vi "_Validate Tune Property.vi"(6 "ConfigRow #":i32, 7 "User Value":dbl=1.0, 8 "Method In":T1={"Lenses"=[], "Mass Ranges"=[], "Acquire"=FALSE, "MCA"=FALSE, "Q1DC EN"=FALSE, "Q1 POL"=FALSE, "Q3 POL"=FALSE, "Q1 RF  EN"=FALSE, "Averaging"=FALSE, "Log Scale"=FALSE, "CPS"=FALSE, "Unit"=FALSE, "Data Path"=path "", "Run Mode"=enum."MRM (Q1/Q2)", "Fixed Mass (amu)"=1.0, "Q3DC EN"=FALSE, "Q3 RF  EN"=FALSE, "Negative"=FALSE} {"Mass Ranges"."Res" items=["High/High", "Medium/Medium", "Low/Low", "High/Medium", "High/Low", "Medium/High", "Medium/Low", "Low/High", "Low/Medium"]}) -> (0 "Lens Table":string[][](table), 1 "DAC Value Out":i32=1, 2 "User Value Out":dbl=1.0, 3 "Method Out":T1={"Lenses"=[], "Mass Ranges"=[], "Acquire"=FALSE, "MCA"=FALSE, "Q1DC EN"=FALSE, "Q1 POL"=FALSE, "Q3 POL"=FALSE, "Q1 RF  EN"=FALSE, "Averaging"=FALSE, "Log Scale"=FALSE, "CPS"=FALSE, "Unit"=FALSE, "Data Path"=path "", "Run Mode"=enum."MRM (Q1/Q2)", "Fixed Mass (amu)"=1.0, "Q3DC EN"=FALSE, "Q3 RF  EN"=FALSE, "Negative"=FALSE} {"Mass Ranges"."Res" items=["High/High", "Medium/Medium", "Low/Low", "High/Medium", "High/Low", "Medium/High", "Medium/Low", "Low/High", "Low/Medium"]})   [LabVIEW 2012]
uses:
  Type/_GUI Method.ctl
  Type/_Lens Property.ctl
  Type/_Mass Range Property.ctl
  Type/_Mass Range Parameters.ctl
  Type/_RT Res Type.ctl
  Type/_Run Mode.ctl
  _Global Configuration.vi
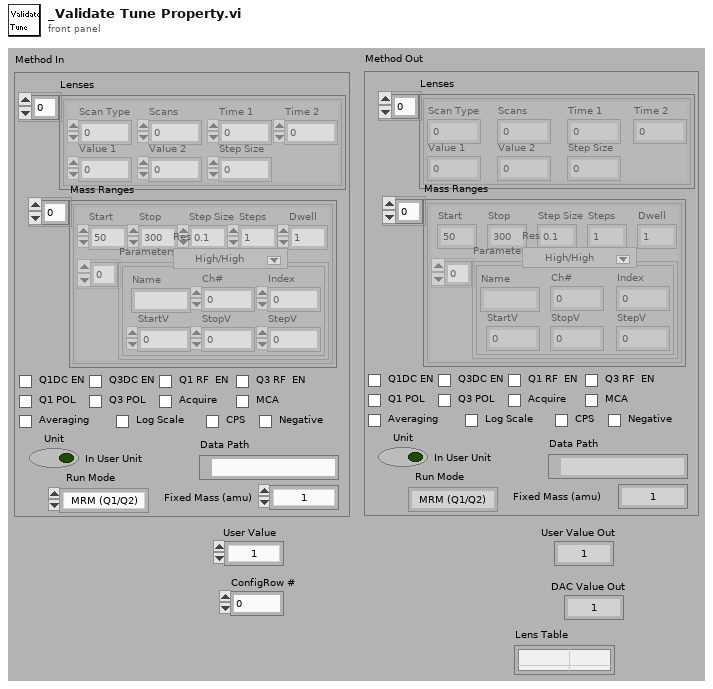
[diagram p1: front panel]
types:
  T1 = typedef "_GUI Method.ctl" = cluster{"Lenses":T2[], "Mass Ranges":T3[], "Acquire":bool, "MCA":bool, "Q1DC EN":bool, "Q1 POL":bool, "Q3 POL":bool, "Q1 RF  EN":bool, "Averaging":bool, "Log Scale":bool, "CPS":bool, "Unit":bool, "Data Path":path, "Run Mode":T6, "Fixed Mass (amu)":dbl, "Q3DC EN":bool, "Q3 RF  EN":bool, "Negative":bool}
  T2 = typedef "_Lens Property.ctl" = cluster{"Scan Type":u8, "Scans":i32, "Time 1":dbl, "Time 2":dbl, "Value 1":dbl, "Value 2":dbl, "Step Size":dbl}
  T3 = typedef "_Mass Range Property.ctl" = cluster{"Start":dbl, "Stop":dbl, "Step Size":dbl, "Steps":i32, "Dwell":dbl, "Parameters":T4[], "Res":T5}
  T4 = typedef "_Mass Range Parameters.ctl" = cluster{"Name":string, "Ch#":u8, "StartV":dbl, "StopV":dbl, "StepV":dbl, "Index":u8}
  T5 = typedef "_RT Res Type.ctl" = u16
  T6 = typedef "_Run Mode.ctl" = enum16{"MRM (Q1/Q2)", "Q1 Scan", "Q1 SRM", "Q2 Scan", "Q2 SRM", "Product Scan", "Precursor Scan", "Neutral Loss", "Neutral Gain"}
  T7 = typedef "_RT Instrument 2.ctl" = cluster{"Table":T8[], "Instrument":string[]}
  T8 = typedef "_RT Configuration 2.ctl" = cluster{"Name":string, "Ch#":u8, "Min":dbl, "Max":dbl, "Def+":dbl, "Def-":dbl, "Offset":dbl, "Slope":dbl, "Type":u8, "Description":string, "SettleT":dbl}
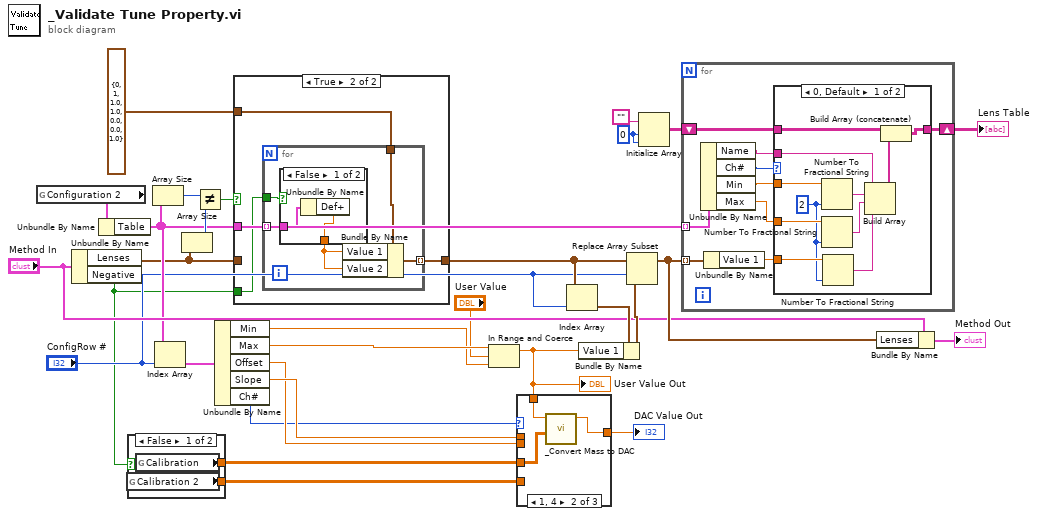
[diagram p0: block diagram]
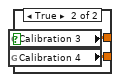
[diagram p2: hidden frame]
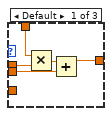
[diagram p3: hidden frame]
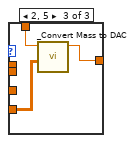
[diagram p4: hidden frame]
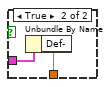
[diagram p6: hidden frame]
diagram:
  w7 = 0 ("dimension size")
  n1 = global read "_Global Configuration.vi" "Configuration 2"() -> (w25:T7)
  n2 = Unbundle By Name("Method In") -> ("Lenses"=w14:T2[], "Negative"=w1:bool)
  n3 = Unbundle By Name(w25) -> ("Table"=w15:T8[])
  n4 = case shown="False" w1 {
    tunnel: [w32 w34] -> w4
    tunnel: [w31 w33] -> w3
    frame False {
      n5 = global read "_Global Configuration.vi" "Calibration 2"() -> (w31:dbl[][])
      n6 = global read "_Global Configuration.vi" "Calibration"() -> (w32:dbl[][])
    }
    frame True {
      n7 = global read "_Global Configuration.vi" "Calibration 3"() -> (w34:dbl[][])
      n8 = global read "_Global Configuration.vi" "Calibration 4"() -> (w33:dbl[][])
    }
  }
  n9 = Array Size(array=w15) -> (size(s)=w18:i32)
  n10 = Index Array(array=w15, index="ConfigRow #") -> (element=w24:T8)
  n11 = Array Size(array=w14) -> (size(s)=w19:i32)
  n12 = Not Equal?(x=w18, y=w19) -> (x != y?=w17:bool)
  n13 = Unbundle By Name(w24) -> ("Min"=w27:dbl, "Max"=w28:dbl, "Offset"=w29:dbl, "Slope"=w30:dbl, "Ch#"=w26:u8)
  n14 = case shown="True" w17 {
    tunnel: w15 -> [_ w39]
    tunnel: w14 -> [w35 _]
    tunnel: [w35 w38] -> w13
    tunnel: T2 {"Scan Type"=0, "Scans"=1, "Time 1"=1.0, "Time 2"=1.0, "Value 1"=0.0, "Value 2"=0.0, "Step Size"=1.0} ("Lenses") -> [_ w37]
    tunnel: w1 -> [_ w36]
    frame False {
    }
    frame True {
      n15 = for {
        tunnel: w39 -> [w43] mode=indexing
        tunnel: w37 -> [w44]
        tunnel: [w41] -> w38 mode=indexing
        tunnel: w36 -> [w40]
        n16 = case shown="False" w40 {
          tunnel: w43 -> [w46 w48]
          tunnel: [w45 w47] -> w42
          frame False {
            n17 = Unbundle By Name(w46) -> ("Def+"=w45:dbl)
          }
          frame True {
            n18 = Unbundle By Name(w48) -> ("Def-"=w47:dbl)
          }
        }
        n19 = Bundle By Name(cluster=w44, "Value 1"=w42, "Value 2"=w42) -> (w41:T2)
      }
    }
  }
  n20 = In Range and Coerce(upper limit=w28, x="User Value", lower limit=w27) -> (coerced(x)=w9:dbl)  [unwired: 1 out]
  "User Value Out" <- w9
  n21 = case shown="1, 4" w26 {
    tunnel: w9 -> [w52 w56 w59]
    tunnel: [w49 w55 w58] -> w10
    tunnel: w30 -> [w51 _ _]
    tunnel: w29 -> [w50 _ _]
    tunnel: w4 -> [_ w54 _]
    tunnel: w3 -> [_ _ w57]
    frame Default {
      n22 = Multiply(x=w52, y=w51) -> (x*y=w53:dbl)
      n23 = Add(x=w53, y=w50) -> (x+y=w49:dbl)
    }
    frame 1, 4 {
      n24 = call "_Convert Mass to DAC.vi"("Calibration Table"=w54, "Mass"=w56) -> ("DAC Value"=w55:dbl)  [unwired: 2 in, 3 out]
    }
    frame 2, 5 {
      n25 = call "_Convert Mass to DAC.vi"("Calibration Table"=w57, "Mass"=w59) -> ("DAC Value"=w58:dbl)  [unwired: 2 in, 3 out]
    }
  }
  "DAC Value Out" <- w10
  n26 = Index Array(array=w13, index="ConfigRow #") -> (element=w23:T2)
  n27 = Bundle By Name(cluster=w23, "Value 1"=w9) -> (w22:T2)
  n28 = Replace Array Subset(array=w13, new element=w22, index="ConfigRow #") -> (w21:T2[])
  n29 = Initialize Array("", w7, w7) -> (w8:string[][])
  n30 = for {
    tunnel: w21 -> [w65] mode=indexing
    tunnel: w15 -> [w66] mode=indexing
    shift-right: [w60] -> w5
    shift-left: w8 -> [w61]
    n31 = Unbundle By Name(w66) -> ("Name"=w63:string, "Ch#"=w62:u8, "Min"=w67:dbl, "Max"=w68:dbl)
    n32 = Unbundle By Name(w65) -> ("Value 1"=w64:dbl)
    n33 = case shown="0, Default" w62 {
      tunnel: w68 -> [w79 _]
      tunnel: w67 -> [w78 _]
      tunnel: [w69 w80] -> w60
      tunnel: w64 -> [w75 _]
      tunnel: w63 -> [w72 _]
      tunnel: w61 -> [w71 w80]
      frame 0, Default {
        w74 = 2
        n34 = Number To Fractional String(number=w78, precision (6)=w74) -> (F-format string=w73:string)  [unwired: 2 out]
        n35 = Number To Fractional String(number=w79, precision (6)=w74) -> (F-format string=w77:string)  [unwired: 2 out]
        n36 = Number To Fractional String(number=w75, precision (6)=w74) -> (F-format string=w76:string)  [unwired: 2 out]
        n37 = Build Array(w72, w73, w77, w76) -> (w70:string[])
        n38 = Build Array (concatenate)(w71, w70) -> (w69:string[][])
      }
      frame 1, 2, 4, 5, 7, 9 {
      }
    }
  }
  "Lens Table" <- w5
  n39 = Bundle By Name(cluster="Method In", "Lenses"=w21) -> (→"Method Out":T1)
